vi "Selection Changed CallBack VI.vi"(4 "Message":refnum<vi>, 5 "事件数据":cluster{"sender":refnum<k24>, "e":refnum<k24>}, 6 "控件引用":refnum<k24>, 7 "事件通用数据":cluster{"事件源":i32, "事件类型":u32, "时间标识":u32}) -> ()   [LabVIEW 2012]
uses:
  System.Windows.Forms
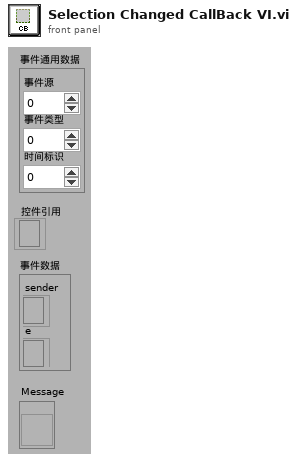
[diagram p1: front panel]
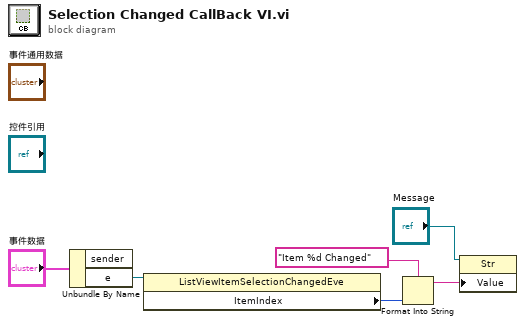
[diagram p0: block diagram]
diagram:
  n1 = Unbundle By Name("事件数据") -> ("e"=w5:refnum<k24>)  [unwired: 1 out]
  n2 = property class="ListViewItemSelectionChangedEve"(reference=w5) -> ("ItemIndex"=w2:i32)  [unwired: 1 in, 2 out]
  n3 = Format Into String(format string="Item %d Changed" ("格式字符串"), w2) -> (resulting string=w1:string)  [unwired: 2 in, 1 out]
  n4 = property class="Str"(reference="Message", "Value"=w1) -> ()  [unwired: 1 in, 2 out]
